vi "Configure Detector Mode.vi"(8 "error in (no error)":errorcluster, 10 "Detector Mode":T1(ring), 11 "SA-ESA in":refnum<class "SA-ESA.lvclass">) -> (0 "error out":errorcluster, 3 "SA-ESA out":refnum<class "SA-ESA.lvclass">)   [LabVIEW 2020, in "SA-ESA.lvclass"]
doc: "Sets the detector mode for the ESA spectrum analyzer.\nOnly Positive Peak. Negative Peak, RMS and Average are supported."
uses:
  SA-ESA.lvclass
  C:/Sandbox/RF Bench/Source Code/WiSpry Test Framework/Instruments/Instrument.lvclass
  Instrument.lvclass/Instrument.ctl
  Instrument.lvclass
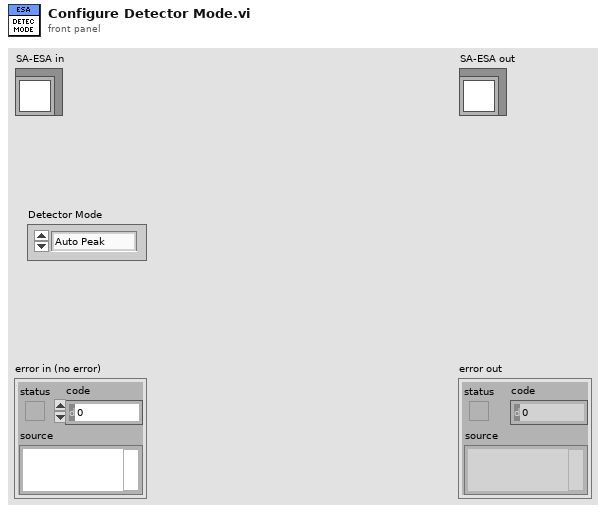
[diagram p1: front panel]
types:
  T1 = enum16{"Auto Peak", "Negative Peak", "Positive Peak", "Quasipeak", "Sample", "RMS", "Average", "CISPR Average", "CISPR RMS"}
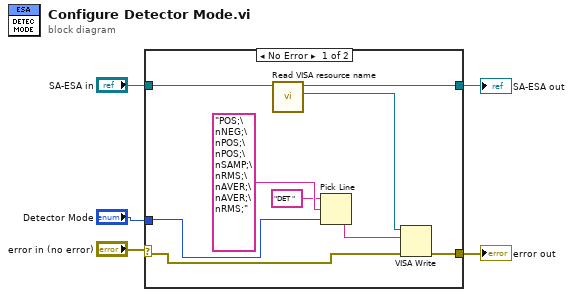
[diagram p0: block diagram]
diagram:
  n1 = case shown="No Error" "error in (no error)" {
    selector: "error in (no error)" -> [w9 w15]
    tunnel: "SA-ESA in" -> [w14 w16]
    tunnel: "Detector Mode" -> [w11 _]
    tunnel: [w7 w16] -> w2
    tunnel: [w6 w15] -> w1
    frame No Error {
      n2 = call "Read VISA resource name.vi"("Instrument in"=w14) -> ("VISA resource name"=w8:refnum<visa-resource-name>, "Instrument out"=w7:refnum<class "SA-ESA.lvclass">)  [unwired: 9 in]
      n3 = Pick Line(string ("")="DET ", multi-line string="POS;\nNEG;\nPOS;\nPOS;\nSAMP;\nRMS;\nAVER;\nAVER;\nRMS;", line index=w11) -> (output string=w10:string)
      n4 = VISA Write(VISA resource name=w8, write buffer=w10, error in (no error)=w9) -> (error out=w6:errorcluster)  [unwired: 2 out]
    }
    frame Error {
    }
  }
  "error out" <- w1
  "SA-ESA out" <- w2
